vi "telemetry_subscriber2.vi"() -> ()   [LabVIEW 2016]
uses:
  ts_sallv_exa/DataTypes/Timestamp.ctl
  ts_sallv_exa/SALLV_EXA.lvlib
panel:
  out "Looptime 2":dbl(graph)
  out "Time":T1
  out "Count":i32
  out "Stop 2":bool=TRUE
  out "Stop":bool=TRUE
  in  "stop":bool
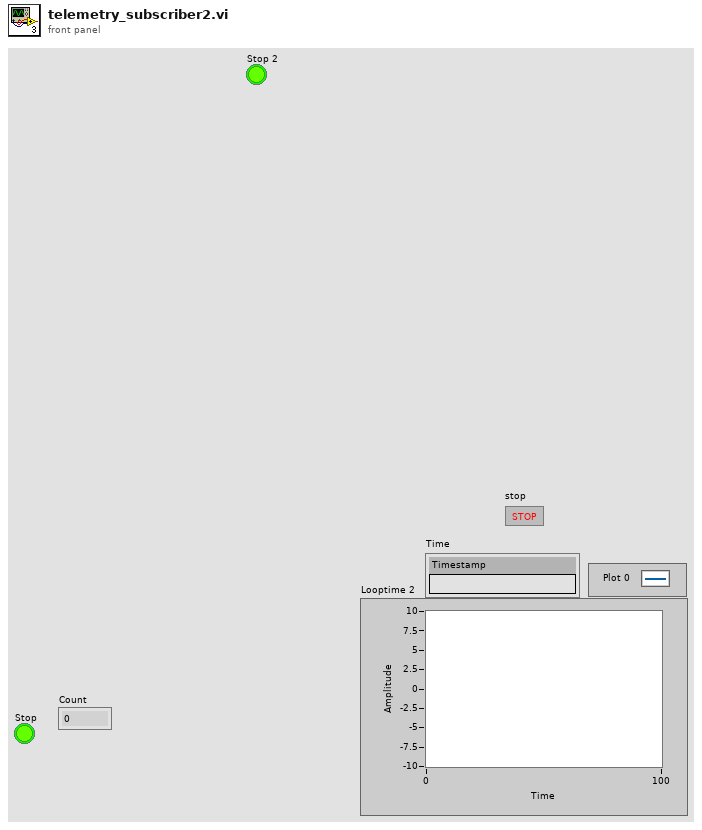
[diagram p1: front panel]
types:
  T1 = typedef "SALLV_EXA.lvlib/Timestamp.ctl" = cluster{"Timestamp":string}
  T2 = typedef "SALLV_EXA.lvlib/LoopTime_ms.ctl" = cluster{"LoopTime_ms":dbl}
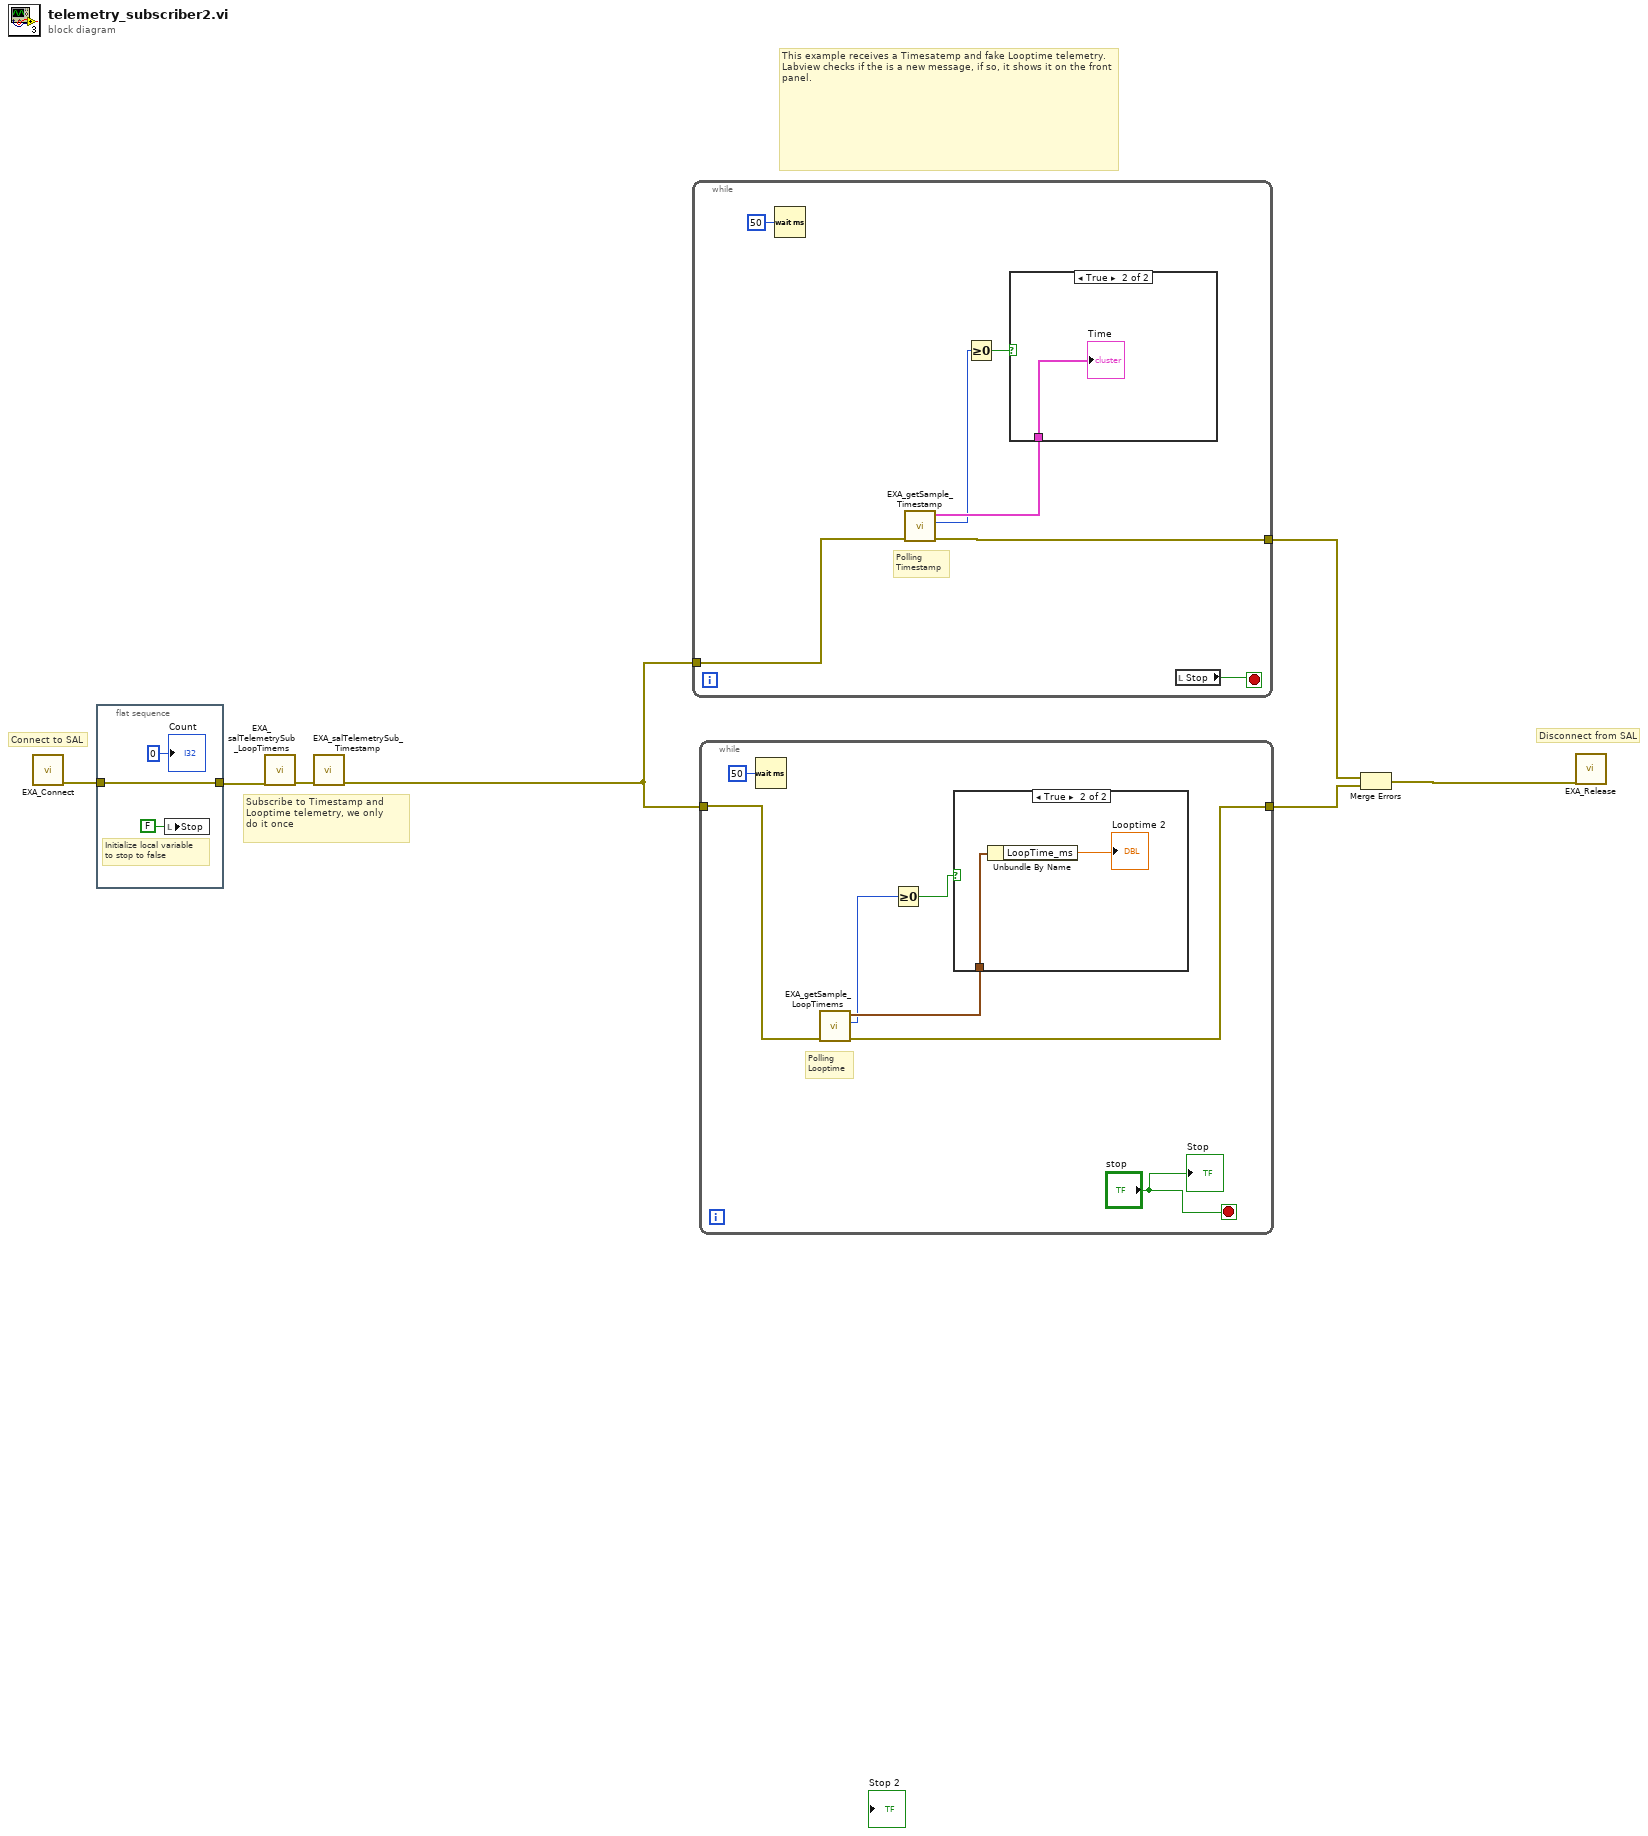
[diagram p0: block diagram]
diagram:
  # "This example receives a Timesatemp and fake Looptime telemetry. Labview checks if the is a new message, if so, it shows it on the front panel."
  # "Subscribe to Timestamp and Looptime telemetry, we only\ndo it once"
  # "Disconnect from SAL"
  # "Connect to SAL"
  n1 = call "EXA_Connect.vi"() -> ("error out"=w7:errorcluster)  [unwired: 10 in, 1 out]
  n2 = flat-sequence {
    tunnel: w7 -> [w9]
    tunnel: [w9] -> w4
    frame #0 {
      # "Initialize local variable \nto stop to false"
      n3 = local write "Stop"(FALSE ("Stop")) -> ()
      "Count" <- 0 ("Count")
    }
  }
  n4 = call "EXA_salTelemetrySub_LoopTimems.vi"("error in (no error)"=w4) -> ("error out"=w5:errorcluster)  [unwired: 9 in, 1 out]
  n5 = call "EXA_salTelemetrySub_Timestamp.vi"("error in (no error)"=w5) -> ("error out"=w1:errorcluster)  [unwired: 9 in, 1 out]
  n6 = while {
    tunnel: w1 -> [w16]
    tunnel: [w15] -> w2
    stop <- w17 stop-if-true
    # "Polling\nTimestamp"
    n7 = Wait (ms)(milliseconds to wait=u32 50) -> ()  [unwired: 1 out]
    n8 = call "EXA_getSample_Timestamp.vi"("error in (no error)"=w16) -> ("error out"=w15:errorcluster, "function return"=w12:i32, "Timestamp_Ctl out"=w14:T1)  [unwired: 8 in]
    n9 = Greater Or Equal To 0?(x=w12) -> (x >= 0?=w13:bool)
    n10 = case shown="True" w13 {
      tunnel: w14 -> [_ w18]
      frame False {
      }
      frame True {
        "Time" <- w18
      }
    }
    n11 = local read "Stop"() -> (w17:bool)
  }
  n12 = while {
    tunnel: w1 -> [w23]
    tunnel: [w22] -> w6
    stop <- "stop" stop-if-true
    # "Polling\nLooptime"
    n13 = Wait (ms)(milliseconds to wait=u32 50) -> ()  [unwired: 1 out]
    n14 = call "EXA_getSample_LoopTimems.vi"("error in (no error)"=w23) -> ("error out"=w22:errorcluster, "function return"=w20:i32, "LoopTime_ms_Ctl out"=w24:T2)  [unwired: 8 in]
    n15 = Greater Or Equal To 0?(x=w20) -> (x >= 0?=w21:bool)
    n16 = case shown="True" w21 {
      tunnel: w24 -> [_ w27]
      frame False {
      }
      frame True {
        n17 = Unbundle By Name(w27) -> ("LoopTime_ms"=→"Looptime 2":dbl)
      }
    }
    "Stop" <- "stop"
  }
  n18 = Merge Errors(w2, w6) -> (w3:errorcluster)
  n19 = call "EXA_Release.vi"("error in (no error)"=w3) -> ()  [unwired: 9 in, 2 out]
